vi "Decorate.vi"(8 "error in (no error)":errorcluster, 10 "Beverage.lvclass":refnum<class "Beverage.lvclass">, 11 "Whip in":refnum<class "Whip.lvclass">) -> (0 "error out":errorcluster, 3 "Whip out":refnum<class "Whip.lvclass">)   [LabVIEW 2013, in "Whip.lvclass"]
uses:
  Whip.lvclass
  Beverage/Beverage.lvclass
  Whip.lvclass/Whip.ctl
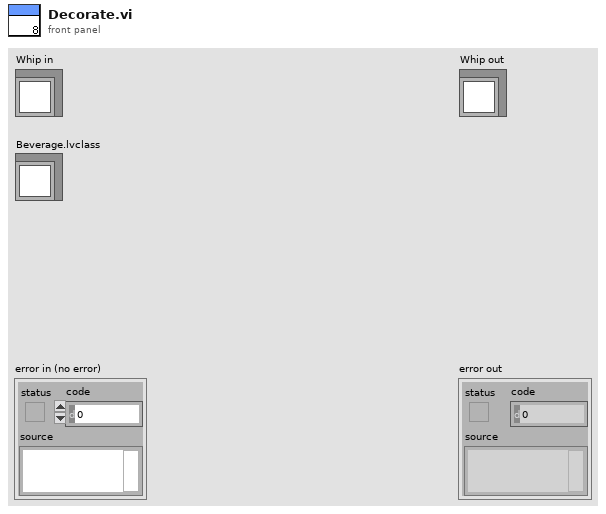
[diagram p1: front panel]
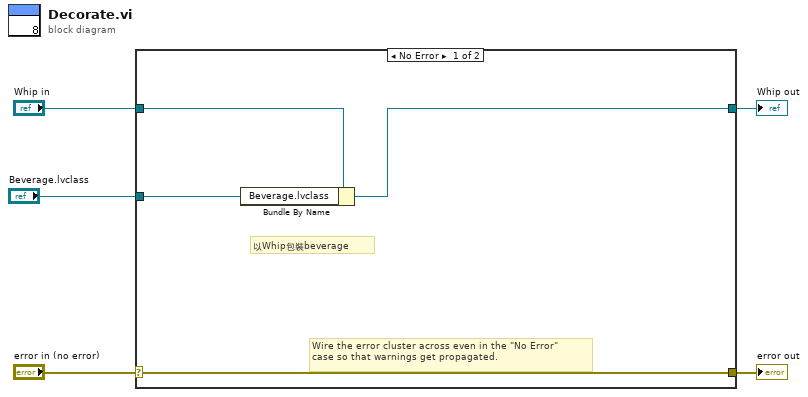
[diagram p0: block diagram]
diagram:
  n1 = case shown="No Error" "error in (no error)" {
    selector: "error in (no error)" -> [w9 w11]
    tunnel: [w9 w11] -> w4
    tunnel: [w6 w10] -> w2
    tunnel: "Whip in" -> [w7 w10]
    tunnel: "Beverage.lvclass" -> [w8 _]
    frame No Error {
      # "以Whip包裝beverage"
      # "Wire the error cluster across even in the \"No Error\"\ncase so that warnings get propagated."
      n2 = Bundle By Name(cluster=w7, "Beverage.lvclass"=w8) -> (w6:refnum<class "Whip.lvclass">)
    }
    frame Error {
    }
  }
  "error out" <- w4
  "Whip out" <- w2
